vi "u8 to Bool.vi"(11 "Input":u8 format="%08b") -> (3 "Output":bool[](array[boolean]))   [LabVIEW 2025, in "TD4.lvclass"]
uses:
  TD4.lvclass
  TD4.lvclass/TD4.ctl
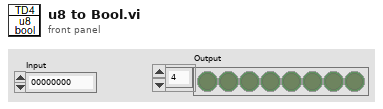
[diagram p1: front panel]
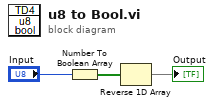
[diagram p0: block diagram]
diagram:
  n1 = Number To Boolean Array(number="Input") -> (Boolean array=w2:bool[])
  n2 = Reverse 1D Array(array=w2) -> (reversed array=→"Output":bool[])
